vi "Default Channel Configuration.vi"() -> (2 "Conversion Time":u16(ring) items=["200 ms", "2.5 ms"], 3 "Degree Range":u8(ring)=2 items=["Raw Ohms", "Degrees Kelvin", "Degrees Celsius", "Degrees Fahrenheit", "Degrees Rankine"], 4 "RTD Types":u8(ring)=1 items=["TCR3851"=1, "TCR3750"=2, "TCR3916"=3, "TCR3920"=4, "TCR3911"=5, "TCR3928"=6, "Custom"=0], 6 "RTD_A":dbl=0.0039083, 8 "RTD_B":dbl=-5.775e-07, 10 "RTD_C":dbl=-4.183e-12, 15 "RTD_Ro":dbl=100.0)   [LabVIEW 2017, in "Modules.lvlib" / "9216.lvclass"]
uses:
  9216.lvclass
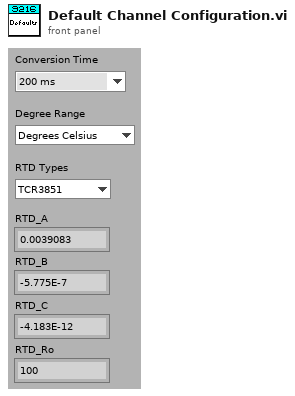
[diagram p1: front panel]
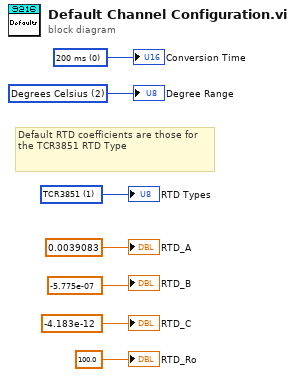
[diagram p0: block diagram]
diagram:
  w1 = u8 1 items=["TCR3851"=1, "TCR3750"=2, "TCR3916"=3, "TCR3920"=4, "TCR3911"=5, "TCR3928"=6, "Custom"=0] ("RTD Type")
  w2 = u8 2 items=["Raw Ohms", "Degrees Kelvin", "Degrees Celsius", "Degrees Fahrenheit", "Degrees Rankine"] ("Temperature Units")
  w3 = u16 0 items=["200 ms", "2.5 ms"] ("Conversion Time")
  # "Default RTD coefficients are those for the TCR3851 RTD Type"
  "RTD_A" <- 0.0039083 ("Numeric")
  "RTD_B" <- -5.775e-07 ("Numeric")
  "RTD_C" <- -4.183e-12 ("Numeric")
  "RTD_Ro" <- 100.0 ("Numeric")
  "Conversion Time" <- w3
  "Degree Range" <- w2
  "RTD Types" <- w1
